vi "gfitsio-create-tbl.vi"(4 "tbltype":T1 items=["ANY_HDU"=-1, "IMAGE_HDU"=0, "ASCII_TBL"=1, "BINARY_TBL"=2], 7 "extname":string, 8 "error in (no error)":errorcluster, 11 "gfits refnum":T2) -> (0 "error out":errorcluster, 3 "dup gfits refnum":T2)   [LabVIEW 2022 SP3, in "gfitsio.lvlib"]
doc: "Create a new ASCII or bintable table extension. The tbltype parameter defines the type of table and can have values of ASCII_TBL or BINARY_TBL. GFITSIO will automatically increase the size of the table as additional rows are written."
uses:
  gfitsio.lvlib
  gfitsio-refnum.ctl
  cfitsio-hdutypes.ctl
  gfitsio.dll
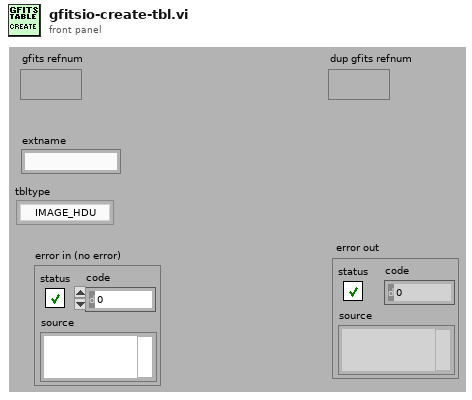
[diagram p1: front panel]
types:
  T1 = typedef "gfitsio.lvlib/cfitsio-hdutypes.ctl" = i32
  T2 = typedef "gfitsio.lvlib/gfitsio-refnum.ctl" = refnum<k1>
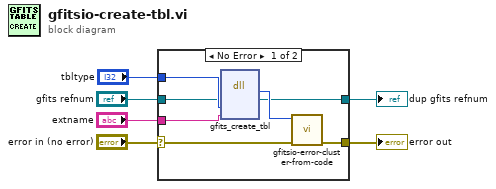
[diagram p0: block diagram]
diagram:
  n1 = case shown="No Error" "error in (no error)" {
    selector: "error in (no error)" -> [w11 w15]
    tunnel: [w13 w15] -> w6
    tunnel: "extname" -> [w10 _]
    tunnel: "gfits refnum" -> [w7 w14]
    tunnel: [w8 w14] -> w3
    tunnel: "tbltype" -> [w9 _]
    frame No Error {
      n2 = dll-call lib="C:/Development/rimas/RIMAS/gfitsio/gfitsio.dll" fn="gfits_create_tbl"("gfits refnum"=w7, "tbltype"=w9, "extname"=w10) -> (w12:i32, "gfits refnum"=w8:T2)  [unwired: 5 in, 2 out]
      n3 = call "gfitsio-error-cluster-from-code.vi"("error in (no error)"=w11, "error code"=w12) -> ("error out"=w13:errorcluster)  [unwired: 9 out]
    }
    frame Error {
    }
  }
  "error out" <- w6
  "dup gfits refnum" <- w3
